vi "Constructor.vi"(6 "Database_location":path=path "D:/Sgraph_database", 7 "OS_type":string="undefined", 8 "error in (no error)":errorcluster, 9 "File extention":string, 10 "DatabaseType":string, 11 "DBAL in":refnum<class "DBAL.lvclass">) -> (0 "error out":errorcluster, 2 "DBAL_class":refnum<data-value>, 3 "DBAL out":refnum<class "DBAL.lvclass">)   [LabVIEW 2020, in "Sgraph_lib_V1.lvlib" / "DBAL.lvclass"]
doc: "The DBAL constructor will make the first DBAL class instance depending on the required database type as defined in the historian ini file."
uses:
  DBAL.lvclass
  DBAL-BIN.lvclass
  D:/Labview/Sgraph/Sgraph/source/DBAL/DBAL.lvclass
  DBAL-BIN.lvclass/DBAL-BIN.ctl
  DBAL-SQLite.lvclass
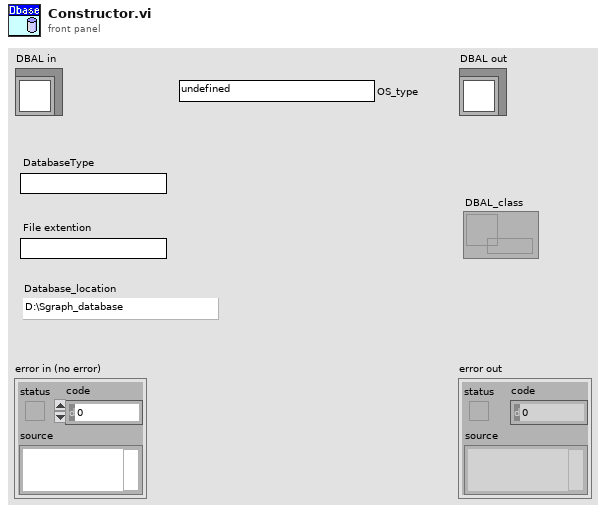
[diagram p1: front panel]
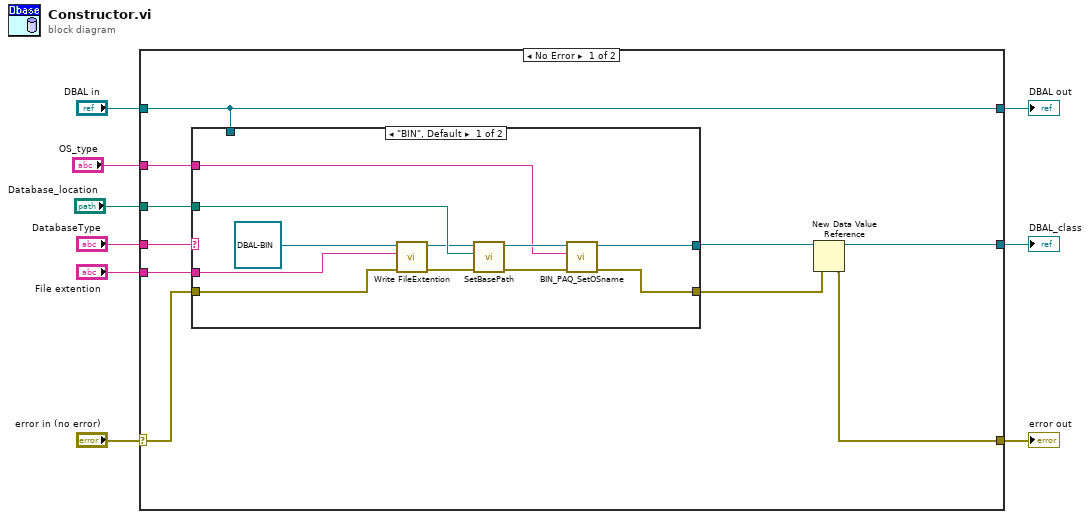
[diagram p0: block diagram]
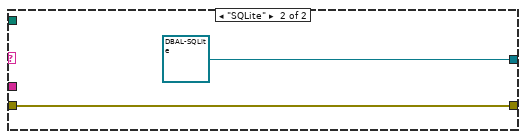
[diagram p2: hidden frame]
diagram:
  n1 = case shown="No Error" "error in (no error)" {
    selector: "error in (no error)" -> [w16 w34]
    tunnel: [w18 w34] -> w8
    tunnel: [w12 w33] -> w6
    tunnel: "DBAL in" -> [w12 w33]
    tunnel: "DatabaseType" -> [w19 _]
    tunnel: [w17 _] -> w4
    tunnel: "File extention" -> [w14 _]
    tunnel: "Database_location" -> [w13 _]
    tunnel: "OS_type" -> [w10 _]
    frame No Error {
      n2 = case shown="\"BIN\", Default" w19 {
        tunnel: [w23 refnum<class "DBAL-SQLite.lvclass"> refnum ("DBAL-SQLite.lvclass")] -> w11
        tunnel: w12 -> [_ _]
        tunnel: w16 -> [w29 w31]
        tunnel: [w21 w31] -> w15
        tunnel: w14 -> [w28 _]
        tunnel: w13 -> [w26 _]
        tunnel: w10 -> [w20 _]
        frame "BIN", Default {
          n3 = call "Write FileExtention.vi"("error in (no error)"=w29, "FileExtention"=w28, "DBAL-BIN in"=refnum<class "DBAL-BIN.lvclass"> refnum ("DBAL-BIN.lvclass")) -> ("error out"=w27:errorcluster, "DBAL-BIN out"=w25:refnum<class "DBAL-BIN.lvclass">)  [unwired: 7 in]
          n4 = call "SetBasePath.vi"("error in (no error)"=w27, "base_path"=w26, "DBAL-BIN in"=w25) -> ("error out"=w22:errorcluster, "DBAL-BIN out"=w24:refnum<class "DBAL-BIN.lvclass">)  [unwired: 7 in]
          n5 = call "BIN_PAQ_SetOSname.vi"("error in (no error)"=w22, "OS_type"=w20, "DBAL-BIN in"=w24) -> ("error out"=w21:errorcluster, "DBAL-BIN out"=w23:refnum<class "DBAL-BIN.lvclass">)  [unwired: 7 in]
        }
        frame "SQLite" {
        }
      }
      n6 = New Data Value Reference(data value=w11, error in=w15) -> (data value reference=w17:refnum<data-value>, error out=w18:errorcluster)
    }
    frame Error {
    }
  }
  "error out" <- w8
  "DBAL out" <- w6
  "DBAL_class" <- w4
